vi "Facade.vi"(0 "Data In":T26 {"Filter"."IIR Filter Cluster"."Forward Coefficients" format="%.4f"; "Filter"."IIR Filter Cluster"."Reverse Coefficients" format="%.4f"}, 2 "Display State In":T24, 3 "Container State":T25) -> (6 "Data Out":T26 {"Filter"."IIR Filter Cluster"."Forward Coefficients" format="%.4f"; "Filter"."IIR Filter Cluster"."Reverse Coefficients" format="%.4f"}, 7 "Display State Out":T24, 8 "Action":T23)   [LabVIEW 2020, in "Multichannel XCtl.xctl"]
uses:
  Multichannel XCtl.xctl
  Data.ctl
  Stimulus Channel XCtl/Stimulus Channel Data.ctl
  Waveform XCtl/Waveform Data.ctl
  Waveform XCtl/Waveform Enum.ctl
  Waveform VIs/Tone VIs/Tone Params.ctl
  Waveform VIs/Pulse Train VIs/Pulse Train Params.ctl
  Waveform VIs/Pulse Train VIs/Pulse Polarity.ctl
  Waveform VIs/Pulse Train VIs/PT-Continuous State.ctl
  Waveform VIs/Noise VIs/Noise Params.ctl
  Waveform VIs/File VIs/StimFile-Params.ctl
  Waveform VIs/FM Sweep VIs/FM Sweep Params.ctl
  Waveform VIs/Chirp Train VIs/Chirp Train.ctl
  Waveform VIs/Chirp Train VIs/Chirp Train Params.ctl
  Waveform VIs/Complex Tone VIs/CT-Params.ctl
  Waveform VIs/Complex Tone VIs/CT-Phase Enum.ctl
  Waveform VIs/Complex Tone VIs/CT-Runtime Data.ctl
  Waveform VIs/Moving Ripple VIs/Moving Ripple.ctl
  Waveform VIs/Moving Ripple VIs/Moving Ripple.Params.ctl
  Waveform VIs/Moving Ripple VIs/Moving Ripple.Data.ctl
  Filter XCtl/Filter Data.ctl
  Gate XCtl/Gate Data.ctl
  Level XCtl/Level Data.ctl
  Level XCtl/Level Units.ctl
  <vilib>/_xctls/Container State.ctl
  State.ctl
  <vilib>/_xctls/Action.ctl
  Stimulus Channel XCtl/Stimulus Channel.xctl
  <vilib>/_xctls/XControlSupport.lvlib
  Gate XCtl/Gate Control.xctl
  Filter XCtl/Filter XCtl.xctl
  Level XCtl/Level XCtl.xctl
  Waveform XCtl/Waveform XCtl.xctl
panel:
  in  "Channel list":i32(listbox)
  in  "Stimulus Params":T22(xcontrol)
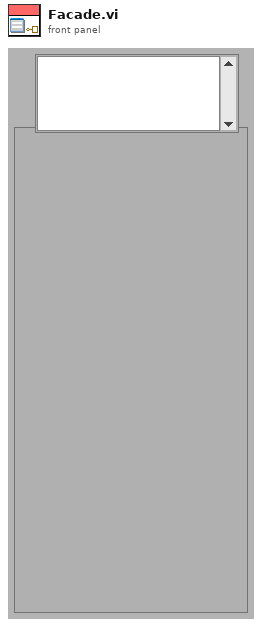
[diagram p1: front panel]
types:
  T1 = typedef "Waveform XCtl.xctl/Waveform Data.ctl" = cluster{"Type":T2, "Tone":T3, "Pulse Train":T4, "Noise":T7, "File":T8, "FMSweep":T9, "Chirp Train":T10, "Complex Tone":cluster{"Params":T12, "Data":T14}, "Moving Ripple":T15}
  T2 = typedef "Waveform Enum.ctl" = enum16{"OFF", "Tone", "Noise", "Pulse Train", "File", "FM Sweep", "Chirp Train", "Complex Tone", "FM Tone", "Moving Ripple"}
  T3 = typedef "Tone Params.ctl" = cluster{"Frequency (kHz)":dbl, "Last Freq":dbl, "Last Phase":dbl}
  T4 = typedef "Pulse Train Params.ctl" = cluster{"Pulse width (us)":dbl, "Pulse rate (Hz)":dbl, "Gap (ms)":dbl, "Polarity":T5, "PT State":T6, "Asynch":bool}
  T5 = typedef "Pulse Polarity.ctl" = enum16{"POS", "NEG", "POS-NEG", "NEG-POS"}
  T6 = typedef "PT-Continuous State.ctl" = cluster{"Template":dbl[], "Nperiod":i32, "Index":i32, "Pulse Rate (Hz)":dbl, "Phase (cycles)":dbl, "Noff":i32}
  T7 = typedef "Noise Params.ctl" = cluster{"InvFilt":bool, "Noise":dbl[], "CurPt":i32, "Aweight":bool, "Seed":i32, "afile":path}
  T8 = typedef "StimFile-Params.ctl" = cluster{"Filename":path, "Signal":dbl[], "Channel":i32, "stream":bool, "offset":i32, "nreps":i32, "loops":i32, "Randomize":bool, "order":i32[], "Seed":i32, "Tokens":i32}
  T9 = typedef "FM Sweep Params.ctl" = cluster{"Rate (oct/s)":dbl, "Fmin (Hz)":dbl, "Fmax (Hz)":dbl, "Ramp (ms)":dbl, "Linear":bool}
  T10 = typedef "Chirp Train.ctl" = cluster{"Params":T11, "Data":cluster{"WF":dbl[]}}
  T11 = typedef "Chirp Train Params.ctl" = cluster{"Fmin (kHz)":dbl, "Fmax (kHz)":dbl, "Compensate":bool, "Duration (ms)":dbl}
  T12 = typedef "CT-Params.ctl" = cluster{"F0 (Hz)":dbl, "Band":cluster{"Flow (Hz)":dbl, "Fhigh (Hz)":dbl}, "Phase":T13, "Min F0 (Hz)":dbl, "Max F0 (Hz)":dbl, "ContinRandPhase":bool, "Max peak factor":dbl, "Max mod depth":dbl, "MinHarmNum":i32, "MaxHarmNum":i32, "Level Mode":enum16{"per component", "overall rms"}, "% jitter":dbl}
  T13 = typedef "CT-Phase Enum.ctl" = enum16{"Cosine", "Random", "Alternating"}
  T14 = typedef "CT-Runtime Data.ctl" = cluster{"Ncomp":i32, "MinHarm":i32, "Phase":dbl[], "Amplitude":dbl[], "Npts/frame":i32, "Last F0":dbl, "Fmin":dbl, "Fmax":dbl, "Lslope":dbl, "randphase":bool, "overall rms":bool, "fmult":dbl[], "jittered":bool}
  T15 = typedef "Moving Ripple.ctl" = cluster{"Params":T16, "Data":T17}
  T16 = typedef "Moving Ripple.Params.ctl" = cluster{"Fmin":dbl, "Fmax":dbl, "Density":dbl, "Velocity":dbl, "Depth":dbl, "Phase":dbl, "Comp/oct":i32}
  T17 = typedef "Moving Ripple.Data.ctl" = cluster{"Freq":dbl[], "A":dbl[], "phase":dbl[], "Phase":dbl}
  T18 = typedef "Filter XCtl.xctl/Filter Data.ctl" = cluster{"CF (kHz)":dbl, "BW (kHz)":dbl, "IIR Filter Cluster":cluster{"filter structure":enum32{"IIR 2nd Order", "IIR 4th Order"}, "Reverse Coefficients":dbl[], "Forward Coefficients":dbl[]}, "Final Filter State":dbl[], "Scale Factor":dbl, "Final Filter State 2":dbl[], "Quadrature":bool, "Type":enum16{"Lowpass", "Highpass", "Bandpass", "Bandstop", "OFF"}}
  T19 = typedef "Gate Control.xctl/Gate Data.ctl" = cluster{"Active":bool, "Delay (ms)":dbl, "Width (ms)":dbl, "Ramp (ms)":dbl}
  T20 = typedef "Level XCtl.xctl/Level Data.ctl" = cluster{"Level":dbl, "Units":T21, "Max":dbl, "Multiplier":dbl, "Cal File":path, "Cal":cluster{"Freq (Hz)":dbl[], "Mag (dB SPL)":dbl[], "Phase (deg)":dbl[]}}
  T21 = typedef "Level Units.ctl" = enum16{"dB atten", "dB SPL", "dB re 1 Vrms", "dB V/Hz½", "mW", "dB HL", "Volts", "dB mW"}
  T22 = cluster{"Waveform":T1, "Filter":T18, "Gate":T19, "Level":T20}
  T23 = typedef "XControlSupport.lvlib/Action.ctl" = cluster{"Data Changed?":bool, "State Changed?":bool, "Action Name":string}
  T24 = typedef "Multichannel XCtl.xctl/State.ctl" = cluster{"names":string[], "Reinit?":bool}
  T25 = typedef "XControlSupport.lvlib/Container State.ctl" = cluster{"Indicator?":bool, "Run Mode?":bool, " Refnum":refnum<vi>}
  T26 = typedef "Multichannel XCtl.xctl/Data.ctl" = T27[]
  T27 = typedef "Stimulus Channel.xctl/Stimulus Channel Data.ctl" = cluster{"Waveform":T1, "Filter":T18, "Gate":T19, "Level":T20}
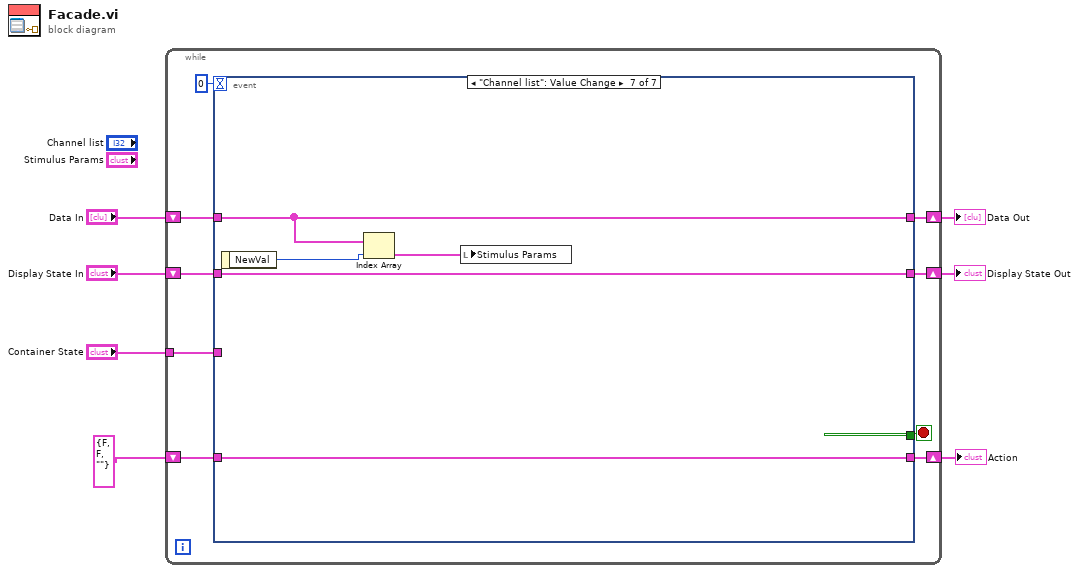
[diagram p0: block diagram]
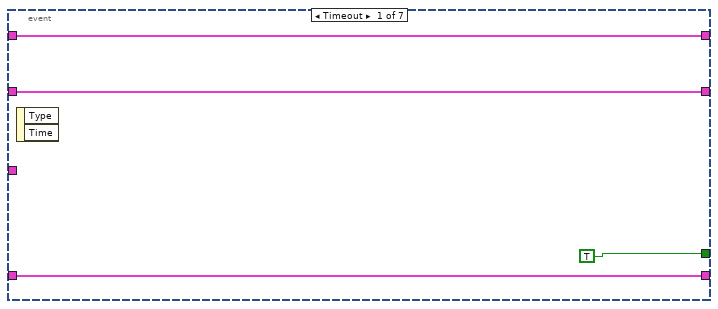
[diagram p2: hidden frame]
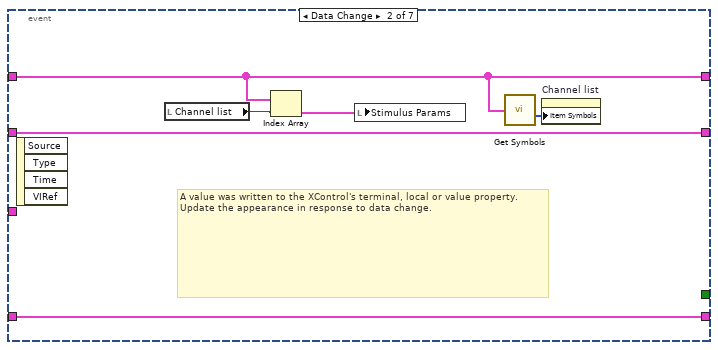
[diagram p3: hidden frame]
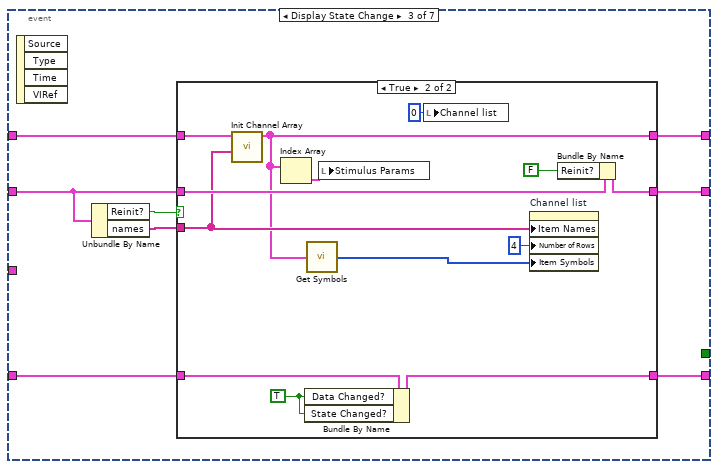
[diagram p4: hidden frame]
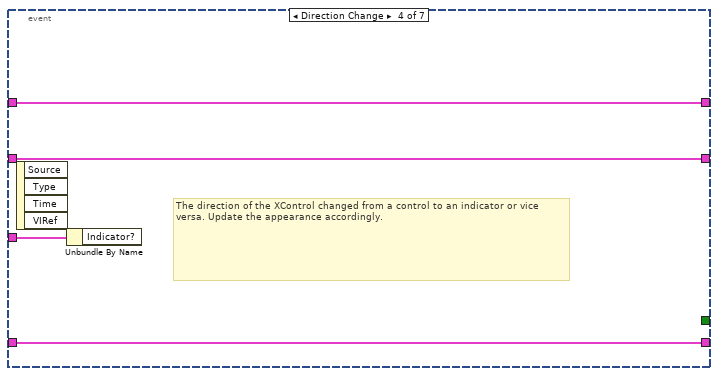
[diagram p6: hidden frame]
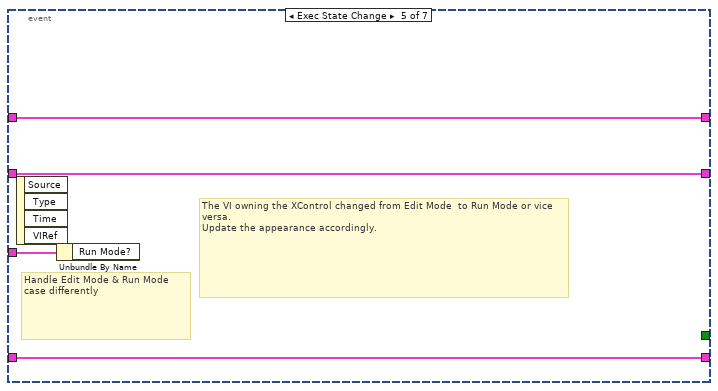
[diagram p7: hidden frame]
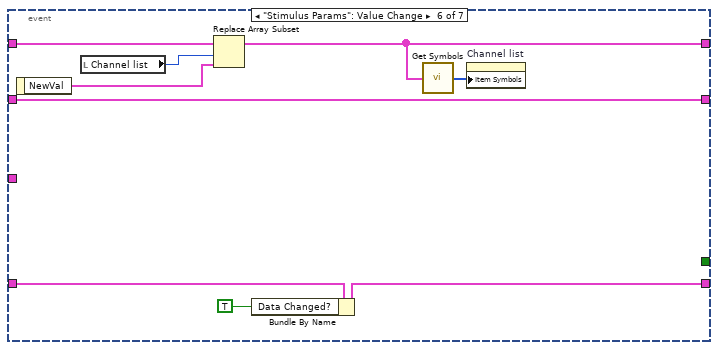
[diagram p8: hidden frame]
diagram:
  n1 = while {
    shift-right: [w15] -> w4
    shift-left: "Display State In" -> [w16]
    tunnel: "Container State" -> [w12]
    shift-right: [w10] -> w7
    shift-left: "Data In" -> [w11]
    shift-right: [w8] -> w2
    shift-left: T23 {"Data Changed?"=FALSE, "State Changed?"=FALSE, "Action Name"=""} ("Action") -> [w9]
    stop <- w14 stop-if-true
    n2 = event shown="[6] \"Channel list\": Value Change" {
      selector: _ -> [_ _ _ _ _ _ _]
      dyn-events: _ -> [_ _ _ _ _ _ _]
      timeout: 0 -> [_ _ _ _ _ _ _]
      tunnel: w16 -> [w18 w26 w31 w53 w57 w61 w71]
      tunnel: [w18 w26 w30 w53 w57 w61 w71] -> w15
      tunnel: [TRUE _ _ _ _ _ _] -> w14
      tunnel: w12 -> [_ _ _ w54 w58 _ _]
      tunnel: w11 -> [w17 w21 w33 w52 w56 w67 w69]
      tunnel: [w17 w21 w32 w52 w56 w59 w69] -> w10
      tunnel: [w19 w25 w28 w51 w55 w63 w72] -> w8
      tunnel: w9 -> [w19 w25 w29 w51 w55 w64 w72]
      event Timeout {
        n3 = event-data() -> ()  [unwired: 1 in, 2 out]
      }
      event Data Change {
        # "A value was written to the XControl's terminal, local or value property.\nUpdate the appearance in response to data change."
        n4 = event-data() -> ()  [unwired: 1 in, 4 out]
        n5 = local read "Channel list"() -> (w23:i32)
        n6 = Index Array(array=w21, index=w23) -> (element=w24:T27)
        n7 = local write "Stimulus Params"(w24) -> ()
        n8 = call "Get Symbols.vi"("Multichannel"=w21) -> ("Symbols"=w22:i32[])
        n9 = property on="Channel list" class="LstBox (strict)"("Item Symbols"=w22) -> ()  [unwired: 2 in, 2 out]
      }
      event Display State Change {
        n10 = event-data() -> ()  [unwired: 1 in, 4 out]
        n11 = Unbundle By Name(w31) -> ("Reinit?"=w34:bool, "names"=w27:string[])
        n12 = case shown="True" w34 {
          tunnel: w33 -> [w37 w44]
          tunnel: [w37 w39] -> w32
          tunnel: w31 -> [w36 w47]
          tunnel: [w36 w46] -> w30
          tunnel: w29 -> [w35 w50]
          tunnel: [w35 w48] -> w28
          tunnel: w27 -> [_ w42]
          frame False {
          }
          frame True {
            w49 = TRUE ("Data Changed?")
            n13 = call "Init Channel Array.vi"("Names"=w42, "Data In"=w44) -> ("Data out"=w39:T26)  [unwired: 9 in]
            n14 = Index Array(array=w39) -> (element=w40:T27)  [unwired: 1 in]
            n15 = Bundle By Name(cluster=w50, "Data Changed?"=w49, "State Changed?"=w49) -> (w48:T23)
            n16 = call "Get Symbols.vi"("Multichannel"=w39) -> ("Symbols"=w38:i32[])
            n17 = local write "Stimulus Params"(w40) -> ()
            n18 = local write "Channel list"(0 ("Channel list")) -> ()
            n19 = property on="Channel list" class="LstBox (strict)"("Item Names"=w42, "Number of Rows"=u32 4, "Item Symbols"=w38) -> ()  [unwired: 2 in, 2 out]
            n20 = Bundle By Name(cluster=w47, "Reinit?"=FALSE) -> (w46:T24)
          }
        }
      }
      event Direction Change {
        # "The direction of the XControl changed from a control to an indicator or vice versa. Update the appearance accordingly."
        n21 = event-data() -> ()  [unwired: 1 in, 4 out]
        n22 = Unbundle By Name(w54) -> ()  [unwired: 1 out]
      }
      event Exec State Change {
        # "The VI owning the XControl changed from Edit Mode  to Run Mode or vice versa.\nUpdate the appearance accordingly."
        # "Handle Edit Mode & Run Mode\ncase differently"
        n23 = event-data() -> ()  [unwired: 1 in, 4 out]
        n24 = Unbundle By Name(w58) -> ()  [unwired: 1 out]
      }
      event "Stimulus Params": Value Change {
        n25 = event-data() -> ("NewVal"=w65:T22)  [unwired: 1 in]
        n26 = local read "Channel list"() -> (w66:i32)
        n27 = Replace Array Subset(array=w67, new element=w65, index=w66) -> (w59:T26)
        n28 = Bundle By Name(cluster=w64, "Data Changed?"=TRUE) -> (w63:T23)
        n29 = call "Get Symbols.vi"("Multichannel"=w59) -> ("Symbols"=w60:i32[])
        n30 = property on="Channel list" class="LstBox (strict)"("Item Symbols"=w60) -> ()  [unwired: 2 in, 2 out]
      }
      event "Channel list": Value Change {
        n31 = event-data() -> ("NewVal"=w70:i32)  [unwired: 1 in]
        n32 = Index Array(array=w69, index=w70) -> (element=w68:T27)
        n33 = local write "Stimulus Params"(w68) -> ()
      }
    }
  }
  "Display State Out" <- w4
  "Data Out" <- w7
  "Action" <- w2
